vi "BotSpeak_COMWrite.vi"(2 "COM Port":u8(slide)=2 scale=1.0..3.0, 3 "string":string, 4 "Bot Settings":T1) -> (0 "response":string, 1 "Bot Settings 2":T1)   [LabVIEW 2012]
doc: "Writes the specified \"string\" to the specified \"COM Port\"."
uses:
  <userlib>/BotSpeak/VIs/Direct/BotSpeak_Control.ctl
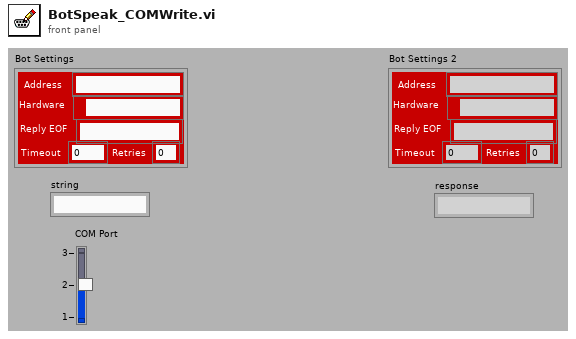
[diagram p1: front panel]
types:
  T1 = typedef "BotSpeak_Control.ctl" = cluster{"Address":string, "Reply EOF":string, "Hardware":path, "Retries":i8, "Timeout":i32}
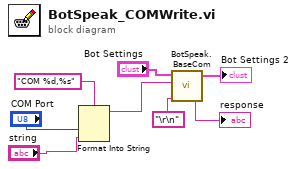
[diagram p0: block diagram]
diagram:
  n1 = Format Into String(format string="COM %d,%s" ("command"), "COM Port", "string") -> (resulting string=w2:string)  [unwired: 2 in, 1 out]
  n2 = call <userlib>:"BotSpeak.BaseCom.vi"("Termination"="\r\n", "command"=w2, "Bot Settings in"="Bot Settings") -> ("response"=→"response":string, "Bot Settings out"=→"Bot Settings 2":T1)  [unwired: 2 in]
